vi "Unsubscribe (SingleTopic).vi"(6 "timeout (100ms)":i32=100, 8 "error in (no error)":errorcluster, 10 "Topic Filter":string, 11 "MQTT_Base in":refnum<class "MQTT_Base.lvclass">) -> (0 "error out":errorcluster, 1 "Ack":bool, 3 "MQTT_Base out":refnum<class "MQTT_Base.lvclass">)   [LabVIEW 2013, in "MQTT Base.lvlib" / "MQTT_Base.lvclass"]
uses:
  MQTT_Base.lvclass
  <vilib>/LabVIEW Open Source Project/MQTT Control Packets/Control Packets/UNSUBSCRIBE/UNSUBSCRIBE.lvclass
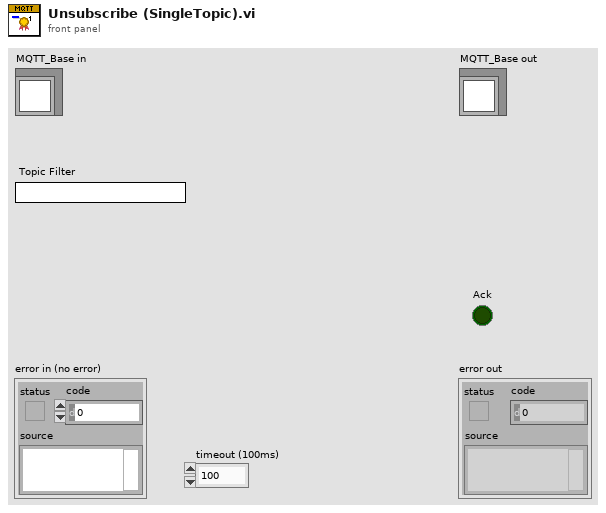
[diagram p1: front panel]
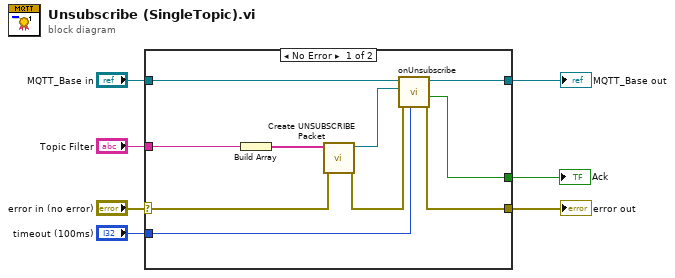
[diagram p0: block diagram]
diagram:
  n1 = case shown="No Error" "error in (no error)" {
    selector: "error in (no error)" -> [w16 w19]
    tunnel: [w11 w19] -> w6
    tunnel: [w10 w18] -> w4
    tunnel: "MQTT_Base in" -> [w14 w18]
    tunnel: "Topic Filter" -> [w15 _]
    tunnel: "timeout (100ms)" -> [w9 _]
    tunnel: [w8 _] -> w1
    frame No Error {
      n2 = Build Array(w15) -> (w17:string[])
      n3 = call <vilib>:"Create UNSUBSCRIBE Packet.vi"("error in (no error)"=w16, "Topic Subscriptions"=w17) -> ("error out"=w12:errorcluster, "UNSUBSCRIBE out"=w13:refnum<class "UNSUBSCRIBE.lvclass">)  [unwired: 7 in, 1 out]
      n4 = call-dynamic "onUnsubscribe.vi"("timeout (100ms)"=w9, "error in (no error)"=w12, "UNSUBSCRIBE"=w13, "MQTT_Base in"=w14) -> ("error out"=w11:errorcluster, "Ack"=w8:bool, "MQTT_Base out"=w10:refnum<class "MQTT_Base.lvclass">)  [unwired: 4 in, 1 out]
    }
    frame Error {
    }
  }
  "error out" <- w6
  "MQTT_Base out" <- w4
  "Ack" <- w1
